vi "ProgressBar.vi"(8 "Frames/set":i32, 9 "#Sets":i32, 10 "Curren Frame":i32, 11 "Current Set":i32) -> (2 "Progress":u8(slide) scale=0.0..100.0, 3 "?":dbl)   [LabVIEW 2015]
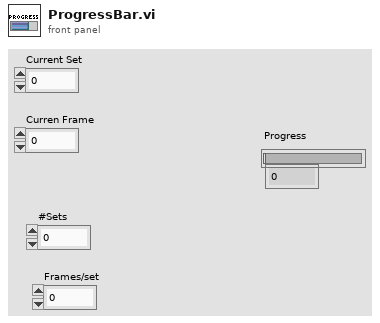
[diagram p1: front panel]
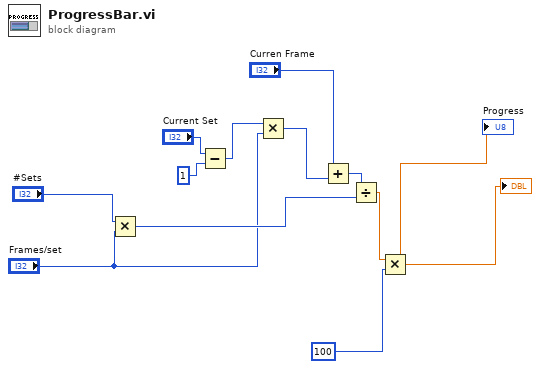
[diagram p0: block diagram]
diagram:
  n1 = Multiply(x="#Sets", y="Frames/set") -> (x*y=w11:i32)
  n2 = Subtract(x="Current Set", y=1) -> (x-y=w1:i32)
  n3 = Multiply(x=w1, y="Frames/set") -> (x*y=w5:i32)
  n4 = Add(x="Curren Frame", y=w5) -> (x+y=w4:i32)
  n5 = Divide(x=w4, y=w11) -> (x/y=w9:dbl)
  n6 = Multiply(x=w9, y=100) -> (x*y=→"Progress" →"?":dbl)
